vi "ASDRestore.vi"(0 "TCP Network Connection Refnum":refnum<k5>, 5 "Restore Flash":bool, 11 "error in (no error)":errorcluster) -> (4 "Header Code":i32, 6 "Error Code":i32, 15 "error out":errorcluster)   [LabVIEW 2010]
panel:
  # "This is a Sub-VI of ASDTCPDemo."
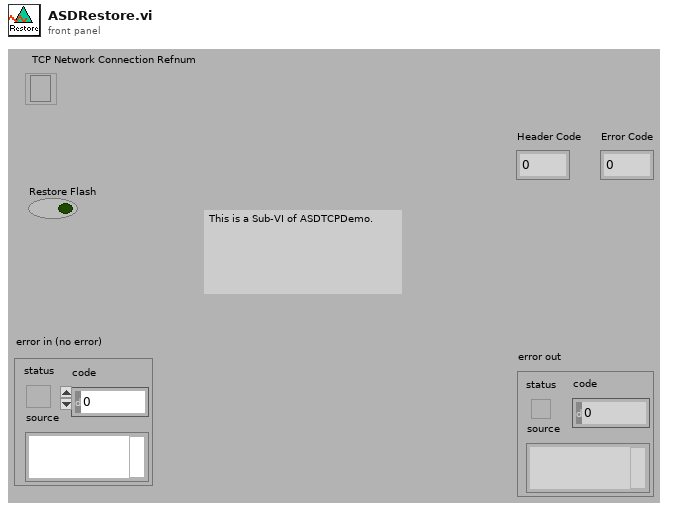
[diagram p1: front panel]
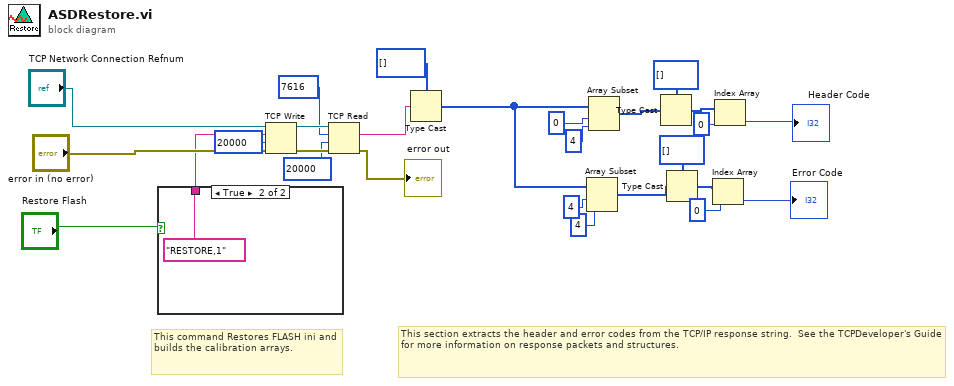
[diagram p0: block diagram]
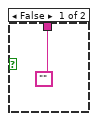
[diagram p2: hidden frame]
diagram:
  # "This section extracts the header and error codes from the TCP/IP response string.  See the TCPDeveloper's Guide for more information on response packets and structures."
  # "This command Restores FLASH ini and builds the calibration arrays."
  n1 = case shown="True" "Restore Flash" {
    tunnel: ["" "RESTORE,1"] -> w20
    frame False {
    }
    frame True {
    }
  }
  n2 = TCP Write(connection ID="TCP Network Connection Refnum", data in=w20, error in (no error)="error in (no error)", 9:20000 ("timeout ms (25000)")) -> (connection ID out=w23:refnum<k5>, error out=w24:errorcluster)  [unwired: 1 out]
  n3 = TCP Read(connection ID=w23, bytes to read=7616, error in (no error)=w24, 9:20000 ("timeout ms (25000)")) -> (data out=w22:string, error out=→"error out":errorcluster)  [unwired: 1 in, 1 out]
  n4 = Type Cast(type=u8[] [], x=w22) -> (*(type *) &x=w11:u8[])
  n5 = Array Subset(array=w11, index=4, length=4 ("index")) -> (w4:u8[])
  n6 = Array Subset(array=w11, index=0 ("start index (0)"), length=4) -> (w10:u8[])
  n7 = Type Cast(type=i32[] [], x=w10) -> (*(type *) &x=w9:i32[])
  n8 = Type Cast(type=i32[] [], x=w4) -> (*(type *) &x=w5:i32[])
  n9 = Index Array(array=w5, index=0) -> (element=→"Error Code":i32)
  n10 = Index Array(array=w9, index=0) -> (element=→"Header Code":i32)
